vi "Test Save Directory.vi"() -> (0 "Reason":string, 1 "Success":bool)   [LabVIEW 2013]
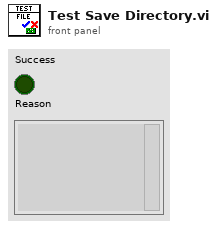
[diagram p1: front panel]
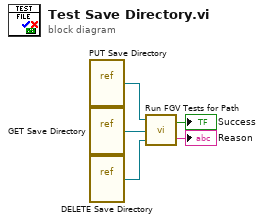
[diagram p0: block diagram]
diagram:
  n1 = vi-ref "PUT Save Directory.vi"() -> (w4:refnum<vi>)
  n2 = vi-ref "GET Save Directory.vi"() -> (w5:refnum<vi>)
  n3 = vi-ref "DELETE Save Directory.vi"() -> (w3:refnum<vi>)
  n4 = call "Run FGV Tests for Path.vi"("DELETE VI Reference"=w3, "GET VI Reference"=w5, "PUT VI Reference"=w4) -> ("Reason"=→"Reason":string, "Success"=→"Success":bool)
